vi "Launch One-Button Dialog Box.vi"(6 "Modal? (T)":bool=TRUE, 7 "Return Msg (Optional)":refnum<class "Dialog Return Msg.lvclass">, 8 "error in (no error)":errorcluster, 9 "Button Text (OK)":string="OK", 10 "Message Text":string) -> (0 "error out":errorcluster)   [LabVIEW 2019, in "OneButtonDialogBox.lvlib" / "OneButtonDialogBox.lvclass"]
uses:
  <vilib>/gpm_packages/@cs/mva-dialogbox/source/OneButtonDialogBox/OneButtonDialogBox.lvclass
  <vilib>/gpm_packages/@cs/mva-dialogbox/source/IDialogBox/IDialogBox Messages/Dialog Return Msg/Dialog Return Msg.lvclass
  <vilib>/gpm_packages/@cs/mva-viewable/Source/IViewable/IViewable/IViewable.lvclass
  C:/Program Files/National Instruments/LabVIEW 2019/vi.lib/ActorFramework/Actor/Actor.lvclass
  C:/Program Files/National Instruments/LabVIEW 2019/vi.lib/gpm_packages/@cs/mva-dialogbox/source/IDialogBox/IDialogBox/IDialogBox.lvclass
  <vilib>/ActorFramework/Actor/Actor.lvclass/Actor.ctl
  <vilib>/ActorFramework/Message Enqueuer/Message Enqueuer.lvclass/Message Enqueuer.ctl
  <vilib>/gpm_packages/@cs/mva-dialogbox/source/OneButtonDialogBox/OneButtonDialogBox.lvclass/OneButtonDialogBox.ctl
  <vilib>/gpm_packages/@cs/mva-dialogbox/source/DialogBoxViewManager/DialogBoxViewManager Messages/Launch Dialog Box Msg/Launch Dialog Box Msg.lvclass/Launch Dialog Box Msg.ctl
  <vilib>/ActorFramework/Message Enqueuer/Init from Existing Queue.vi
  <vilib>/ActorFramework/Message Enqueuer/Enqueue.vi
  <vilib>/gpm_packages/@cs/mva-dialogbox/source/DialogBoxViewManager/DialogBoxViewManager Messages/Launch Dialog Box Msg/Launch Dialog Box Msg.lvclass
  C:/Program Files/National Instruments/LabVIEW 2019/vi.lib/ActorFramework/Message/Message.lvclass
  <vilib>/ActorFramework/Message Priority Queue/Priority Enqueue.vi
  <vilib>/ActorFramework/Message Enqueuer/Message Enqueuer.lvclass
  <vilib>/ActorFramework/Actor/Actor.lvclass
panel:
  in  "Dialog Launcher":refnum<class "IViewable.lvclass">
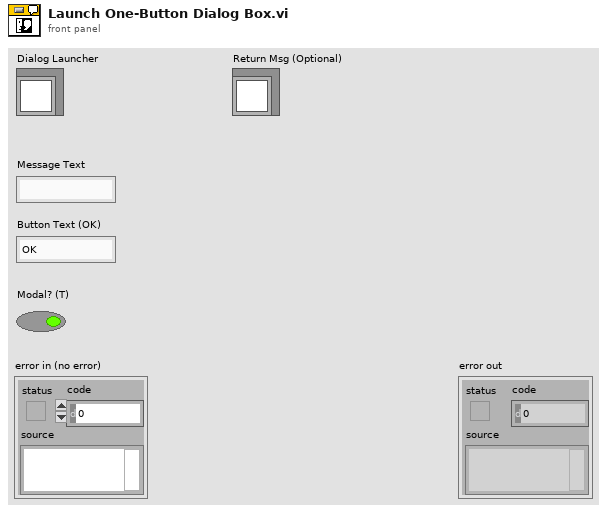
[diagram p1: front panel]
types:
  T1 = enum32{"Invalid", "Default", "Floating", "Floating/Auto-Hide", "Modal"}
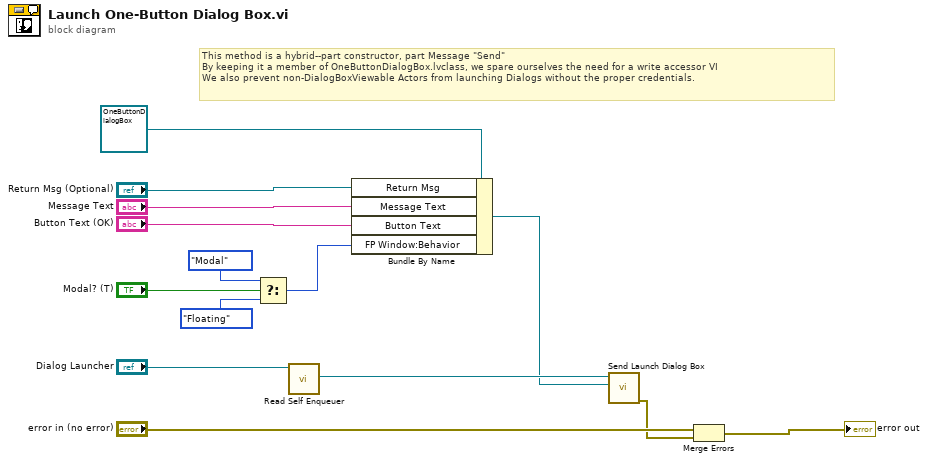
[diagram p0: block diagram]
diagram:
  # "This method is a hybrid--part constructor, part Message \"Send\"\nBy keeping it a member of OneButtonDialogBox.lvclass, we spare ourselves the need for a write accessor VI\nWe also prevent non-DialogBoxViewable Actors from launching Dialogs without the proper credentials."
  n1 = Select(t=T1."Modal" ("FP Window:Behavior"), s="Modal? (T)", f=T1."Floating" ("FP Window:Behavior")) -> (s? t:f=w6:T1)
  n2 = call <vilib>:"Read Self Enqueuer.vi"("Actor"="Dialog Launcher") -> ("Self Enqueuer"=w4:refnum<class "Message Enqueuer.lvclass">)  [unwired: 10 in]
  n3 = Bundle By Name(cluster=refnum<class "OneButtonDialogBox.lvclass"> refnum ("OneButtonDialogBox in"), "Return Msg"="Return Msg (Optional)", "Message Text"="Message Text", "Button Text"="Button Text (OK)", "FP Window:Behavior"=w6) -> (w3:refnum<class "OneButtonDialogBox.lvclass">)
  n4 = call <vilib>:"Send Launch Dialog Box.vi"("DialogBox"=w3, "Message Enqueuer"=w4) -> ("error out"=w1:errorcluster)  [unwired: 8 in, 1 out]
  n5 = Merge Errors("error in (no error)", w1) -> (→"error out":errorcluster)
